vi "8bit-trig.vi"(1 "R":bool, 2 "C":bool, 3 "D cluster":T1) -> (0 "Cluster Q":T2)   [LabVIEW 2017]
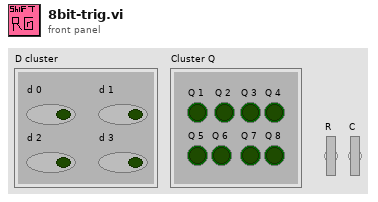
[diagram p1: front panel]
types:
  T1 = cluster{"d 0":bool, "d 1":bool, "d 2":bool, "d 3":bool}
  T2 = cluster{"Q 1":bool, "Q 2":bool, "Q 3":bool, "Q 4":bool, "Q 5":bool, "Q 6":bool, "Q 7":bool, "Q 8":bool}
  T3 = cluster{"q":bool, "q":bool, "q":bool, "q":bool, "q":bool, "q":bool, "q":bool, "q":bool}
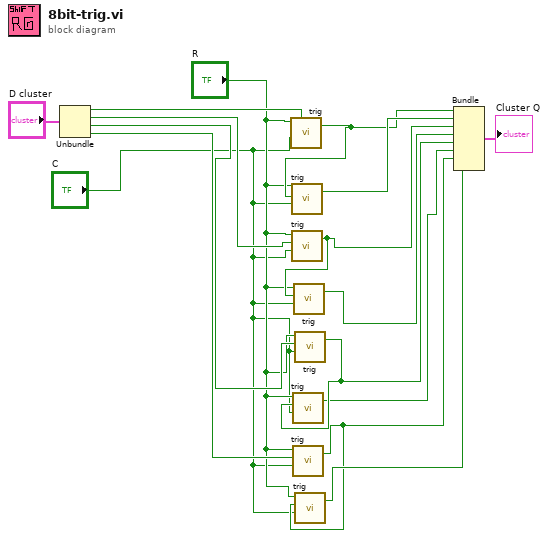
[diagram p0: block diagram]
diagram:
  n1 = Unbundle("D cluster") -> ("d 0"=w12:bool, "d 1"=w9:bool, "d 2"=w6:bool, "d 3"=w13:bool)
  n2 = call "trig.vi"("c"="C", "d"=w12, "r"="R") -> ("q"=w10:bool)  [unwired: 1 in, 1 out]
  n3 = call "trig.vi"("c"="C", "d"=w10, "r"="R") -> ("q"=w11:bool)  [unwired: 1 in, 1 out]
  n4 = call "trig.vi"("c"="C", "d"=w9, "r"="R") -> ("q"=w7:bool)  [unwired: 1 in, 1 out]
  n5 = call "trig.vi"("c"="C", "d"=w13, "r"="R") -> ("q"=w2:bool)  [unwired: 1 in, 1 out]
  n6 = call "trig.vi"("c"="C", "d"=w7, "r"="R") -> ("q"=w8:bool)  [unwired: 1 in, 1 out]
  n7 = call "trig.vi"("c"="C", "d"=w6, "r"="R") -> ("q"=w5:bool)  [unwired: 1 in, 1 out]
  n8 = call "trig.vi"("c"="C", "d"=w5, "r"="R") -> ("q"=w3:bool)  [unwired: 1 in, 1 out]
  n9 = call "trig.vi"("c"="C", "d"=w2, "r"="R") -> ("q"=w15:bool)  [unwired: 1 in, 1 out]
  n10 = Bundle("q"=w10, "q"=w11, "q"=w7, "q"=w8, "q"=w5, "q"=w3, "q"=w2, "q"=w15) -> (→"Cluster Q":T3)  [unwired: 1 in]
